vi "Sweep.vi"(0 "SPU":refnum<k24>, 1 "Refdata_struct":refnum<k24>[](array[refnum]), 2 "TSL":refnum<k24>, 3 "Ref_monitordata_struct":refnum<k24>[](array[refnum]), 4 "PDLSTS":refnum<k24>, 5 "错误输入（无错误）":errorcluster, 7 "PCU":refnum<k24>, 10 "MPM":refnum<k24>[](array[refnum]), 12 "chkeach_ch":bool) -> (19 "错误输出":errorcluster)   [LabVIEW 2017]
doc: "Get Reference"
uses:
  D:/test/PDLSTS/LV_PDL LvVer17.0/LV_PDL_x64/DLL/STSProcess.dll
  DLL/STSProcess.dll
  D:/test/PDLSTS/LV_PDL LvVer17.0/LV_PDL_x64/DLL/InstrumentDLL.dll
  DLL/InstrumentDLL.dll
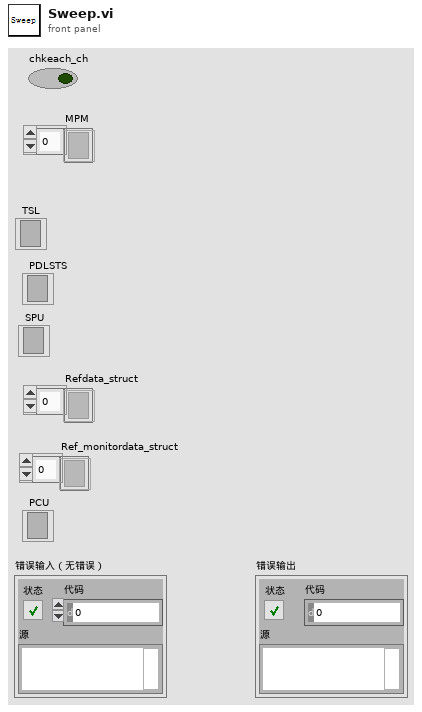
[diagram p1: front panel]
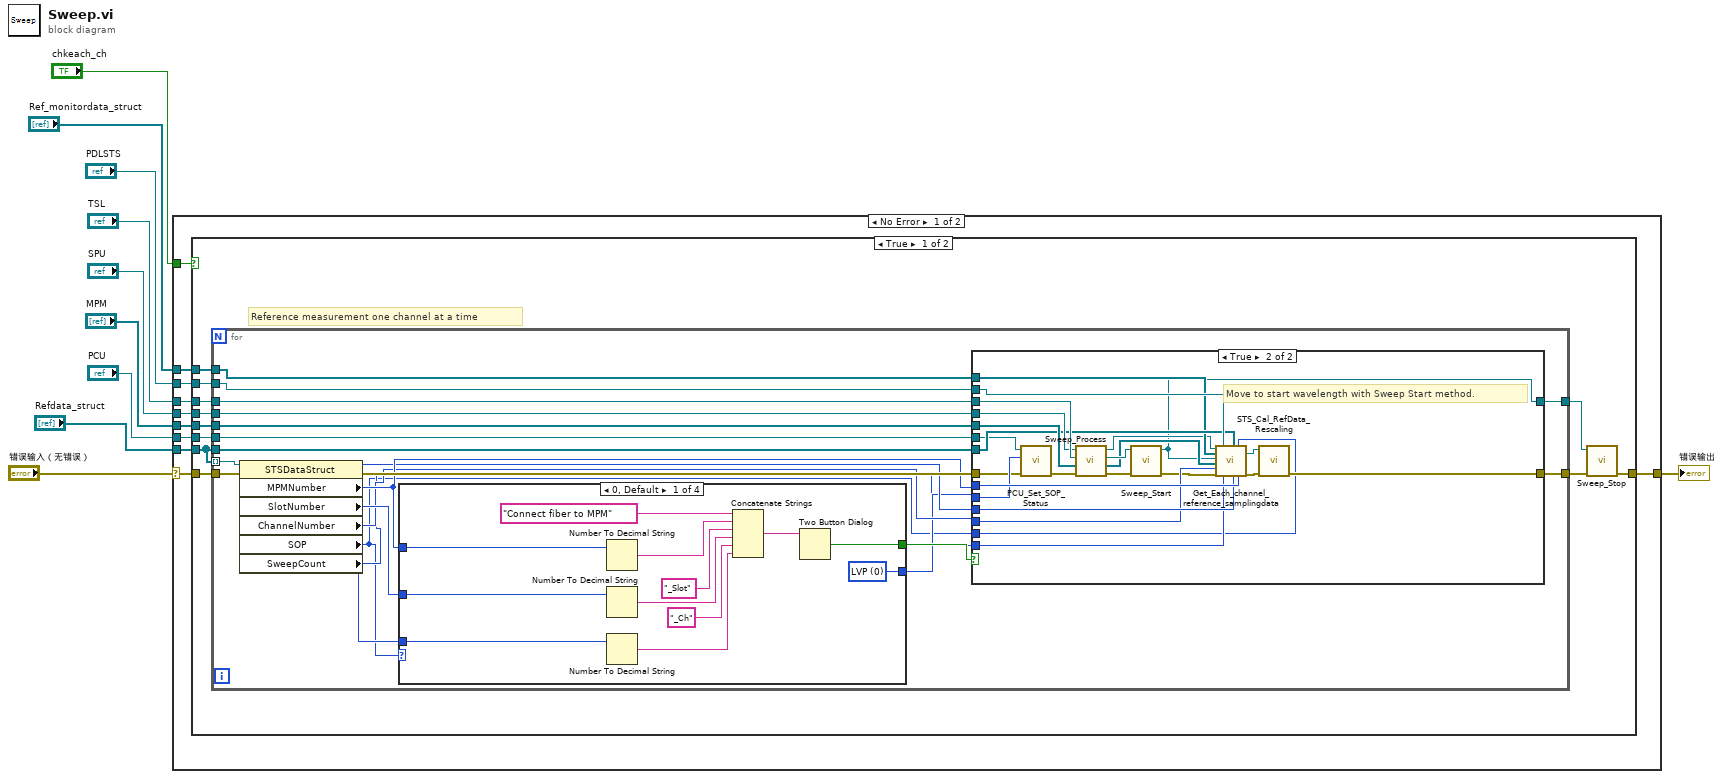
[diagram p0: block diagram]
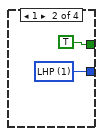
[diagram p2: hidden frame]
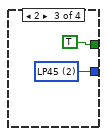
[diagram p3: hidden frame]
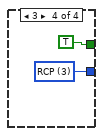
[diagram p4: hidden frame]
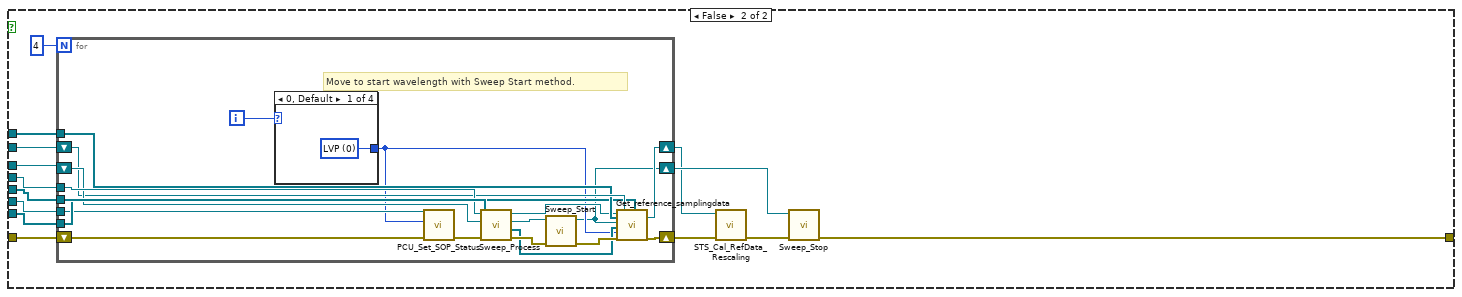
[diagram p6: hidden frame]
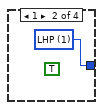
[diagram p7: hidden frame]
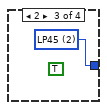
[diagram p8: hidden frame]
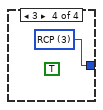
[diagram p9: hidden frame]
diagram:
  n1 = case shown="No Error" "错误输入（无错误）" {
    selector: "错误输入（无错误）" -> [w12 w132]
    tunnel: "Ref_monitordata_struct" -> [w20 _]
    tunnel: "PDLSTS" -> [w19 _]
    tunnel: [w18 w132] -> w9
    tunnel: "SPU" -> [w17 _]
    tunnel: "MPM" -> [w16 _]
    tunnel: "TSL" -> [w15 _]
    tunnel: "chkeach_ch" -> [w14 _]
    tunnel: "Refdata_struct" -> [w13 _]
    tunnel: "PCU" -> [w11 _]
    frame No Error {
      n2 = case shown="True" w14 {
        tunnel: w15 -> [w29 w106]
        tunnel: w16 -> [w31 w108]
        tunnel: w17 -> [w30 w107]
        tunnel: w12 -> [w28 w105]
        tunnel: [w22 w104] -> w18
        tunnel: w13 -> [w25 w101]
        tunnel: w19 -> [w27 w103]
        tunnel: w20 -> [w26 w102]
        tunnel: w11 -> [w21 w95]
        frame True {
          # "Reference measurement one channel at a time"
          n3 = for {
            tunnel: w29 -> [w49]
            tunnel: w31 -> [w47]
            tunnel: w30 -> [w48]
            tunnel: w28 -> [w42]
            tunnel: w25 -> [w41] mode=indexing
            tunnel: w27 -> [w40]
            tunnel: w25 -> [w39]
            tunnel: w26 -> [w38]
            tunnel: [w36] -> w24
            tunnel: [w37] -> w23
            tunnel: w21 -> [w34]
            n4 = property on="属性节点" class="STSDataStruct"(reference=w41, error in=w42) -> (error out=w50:errorcluster, "MPMNumber"=w46:i32, "SlotNumber"=w45:i32, "ChannelNumber"=w44:i32, "SOP"=w32:i32, "SweepCount"=w33:i32)  [unwired: 1 out]
            n5 = case shown="0, Default" w32 {
              tunnel: w46 -> [w55 _ _ _]
              tunnel: w45 -> [w54 _ _ _]
              tunnel: w44 -> [w53 _ _ _]
              tunnel: [w52 TRUE ("T button?") TRUE ("T button?") TRUE ("T button?")] -> w43
              tunnel: [w51 w63 w65 w67] -> w35
              frame 0, Default {
                w51 = 0 items=["LVP", "LHP", "LP45", "RCP", "LN45", "LCP"] ("status")
                n6 = Number To Decimal String(number=w55) -> (decimal integer string=w61:string)  [unwired: 1 in]
                n7 = Number To Decimal String(number=w54) -> (decimal integer string=w59:string)  [unwired: 1 in]
                n8 = Number To Decimal String(number=w53) -> (decimal integer string=w57:string)  [unwired: 1 in]
                n9 = Concatenate Strings("Connect fiber to MPM" ("消息"), w61, "_Slot" ("字符串"), w59, "_Ch" ("字符串"), w57) -> (w56:string)
                n10 = Two Button Dialog(message=w56) -> (T button?=w52:bool)  [unwired: 2 in]
              }
              frame 1 {
                w63 = 1 items=["LVP", "LHP", "LP45", "RCP", "LN45", "LCP"] ("status")
              }
              frame 2 {
                w65 = 2 items=["LVP", "LHP", "LP45", "RCP", "LN45", "LCP"] ("status")
              }
              frame 3 {
                w67 = 3 items=["LVP", "LHP", "LP45", "RCP", "LN45", "LCP"] ("status")
              }
            }
            n11 = case shown="True" w43 {
              tunnel: w50 -> [w70 w76]
              tunnel: w49 -> [w69 w94]
              tunnel: w48 -> [_ w93]
              tunnel: w47 -> [_ w92]
              tunnel: w46 -> [_ w91]
              tunnel: w45 -> [_ w90]
              tunnel: w44 -> [_ w89]
              tunnel: w40 -> [_ w88]
              tunnel: [w70 w78] -> w36
              tunnel: w39 -> [_ w87]
              tunnel: w38 -> [_ w86]
              tunnel: [w69 w71] -> w37
              tunnel: w35 -> [_ w77]
              tunnel: w34 -> [_ w75]
              tunnel: w33 -> [_ w73]
              tunnel: w32 -> [_ w72]
              frame False {
              }
              frame True {
                # "Move to start wavelength with Sweep Start method."
                n12 = call "PCU_Set_SOP_Status.vi"("error in (no error)"=w76, "status"=w77, ".NET Reference in"=w75) -> ("error out"=w74:errorcluster)  [unwired: 7 in, 1 out]
                n13 = call "Sweep_Process.vi"("错误输入（无错误）"=w74, "MPM"=w92, "TSL"=w94, "SPU"=w93) -> ("error out"=w85:errorcluster, "MPM out"=w81:refnum<k24>[], "TSL out"=w82:refnum<k24>, "SPU out"=w80:refnum<k24>)  [unwired: 4 in]
                n14 = call "Sweep_Start.vi"("error in (no error)"=w85, ".NET Reference in"=w82) -> ("error out"=w84:errorcluster, "Reference out"=w71:refnum<k24>)  [unwired: 8 in]
                n15 = call "Get_Each_channel_reference_samplingdata.vi"("SPU"=w80, "Ref_monitordata_struct"=w86, "TSL"=w71, "MPM"=w81, "ChannelNumber"=w89, "错误输入（无错误）"=w84, "STSProcess.PDLSTS"=w88, "SweepCount"=w73, "Refdata_struct"=w87, "SlotNumber"=w90, "SOP"=w72, "MPMNumber"=w91) -> ("PDLSTS out"=w79:refnum<k24>, "error out"=w83:errorcluster)  [unwired: 6 in]
                n16 = call "STS_Cal_RefData_Rescaling.vi"("错误输入（无错误）"=w83, "PDLSTS"=w79) -> ("error out"=w78:errorcluster)  [unwired: 8 in, 1 out]
              }
            }
          }
          n17 = call "Sweep_Stop.vi"("error in (no error)"=w24, ".NET Reference in"=w23) -> ("error out"=w22:errorcluster)  [unwired: 8 in, 1 out]
        }
        frame False {
          n18 = for {
            N: 4 -> [_]
            tunnel: w108 -> [w127]
            tunnel: w107 -> [w126]
            tunnel: w102 -> [w123]
            tunnel: w101 -> [w122]
            shift-right: [w109] -> w99
            shift-left: w106 -> [w125]
            shift-right: [w119] -> w98
            shift-left: w105 -> [w112]
            shift-right: [w115] -> w97
            shift-left: w103 -> [w124]
            tunnel: w95 -> [w113]
            i -> [w114]
            # "Move to start wavelength with Sweep Start method."
            n19 = case shown="0, Default" w114 {
              tunnel: [w128 w129 w130 w131] -> w110
              frame 0, Default {
                w128 = 0 items=["LVP", "LHP", "LP45", "RCP", "LN45", "LCP"] ("status")
              }
              frame 1 {
                w129 = 1 items=["LVP", "LHP", "LP45", "RCP", "LN45", "LCP"] ("status")
                (unwired) TRUE ("T button?")
              }
              frame 2 {
                w130 = 2 items=["LVP", "LHP", "LP45", "RCP", "LN45", "LCP"] ("status")
                (unwired) TRUE ("T button?")
              }
              frame 3 {
                w131 = 3 items=["LVP", "LHP", "LP45", "RCP", "LN45", "LCP"] ("status")
                (unwired) TRUE ("T button?")
              }
            }
            n20 = call "PCU_Set_SOP_Status.vi"("error in (no error)"=w112, "status"=w110, ".NET Reference in"=w113) -> ("error out"=w111:errorcluster)  [unwired: 7 in, 1 out]
            n21 = call "Sweep_Process.vi"("错误输入（无错误）"=w111, "MPM"=w127, "TSL"=w125, "SPU"=w126) -> ("error out"=w121:errorcluster, "MPM out"=w117:refnum<k24>[], "TSL out"=w118:refnum<k24>, "SPU out"=w116:refnum<k24>)  [unwired: 4 in]
            n22 = call "Sweep_Start.vi"("error in (no error)"=w121, ".NET Reference in"=w118) -> ("error out"=w120:errorcluster, "Reference out"=w109:refnum<k24>)  [unwired: 8 in]
            n23 = call "Get_reference_samplingdata.vi"("SPU"=w116, "Ref_monitordata_struct"=w123, "TSL"=w109, "MPM"=w117, "SOP"=w110, "错误输入（无错误）"=w120, "STSProcess.PDLSTS"=w124, "Refdata_struct"=w122) -> ("PDLSTS out"=w115:refnum<k24>, "error out"=w119:errorcluster)  [unwired: 10 in]
          }
          n24 = call "STS_Cal_RefData_Rescaling.vi"("错误输入（无错误）"=w98, "PDLSTS"=w97) -> ("error out"=w100:errorcluster)  [unwired: 8 in, 1 out]
          n25 = call "Sweep_Stop.vi"("error in (no error)"=w100, ".NET Reference in"=w99) -> ("error out"=w104:errorcluster)  [unwired: 8 in, 1 out]
        }
      }
    }
    frame Error {
    }
  }
  "错误输出" <- w9
